vi "PH_DIM.get String.vi"(1 "no link":bool, 2 "typeDescriptor":string, 3 "data":i8[](array[numeric]), 4 "quality":i32) -> (0 "Output String":string)   [LabVIEW 2014, in "PH_Common.lvlib"]
doc: "This VI calculates the status of a string tag. It gives out:\n\nno info available: no link or wrong data type or tag status bad\nelse: link and data type and tag status ok, value = incoming text"
uses:
  PH_Common.lvlib
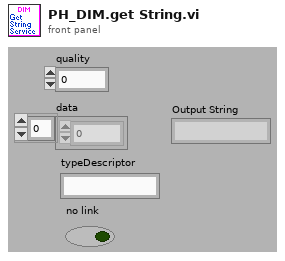
[diagram p1: front panel]
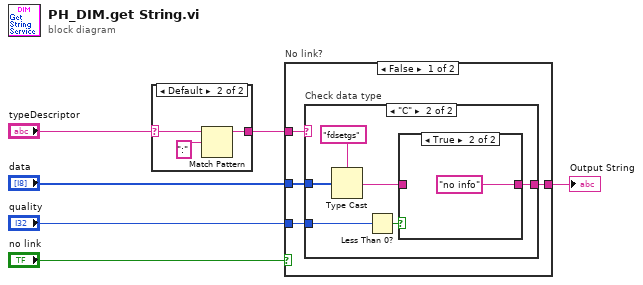
[diagram p0: block diagram]
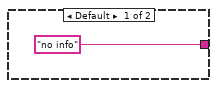
[diagram p3: hidden frame]
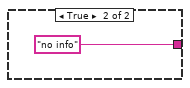
[diagram p5: hidden frame]
diagram:
  n1 = case shown="Default" "typeDescriptor" {
    selector: "typeDescriptor" -> [w7 w8]
    tunnel: [w7 w10] -> w2
    frame "C" {
    }
    frame Default {
      n2 = Match Pattern(string=w8, regular expression=":") -> (before substring=w10:string)  [unwired: 1 in, 3 out]
    }
  }
  n3 = case "No link?" shown="False" "no link" {
    tunnel: [w14 "no info"] -> w6
    tunnel: "quality" -> [w13 _]
    tunnel: "data" -> [w12 _]
    tunnel: w2 -> [w11 _]
    frame False {
      n4 = case "Check data type" shown="\"C\"" w11 {
        tunnel: ["no info" w21] -> w14
        tunnel: w13 -> [_ w19]
        tunnel: w12 -> [_ w18]
        frame Default {
        }
        frame "C" {
          n5 = Type Cast(type="fdsetgs", x=w18) -> (*(type *) &x=w17:string)
          n6 = Less Than 0?(x=w19) -> (x < 0?=w20:bool)
          n7 = case shown="True" w20 {
            tunnel: [w22 "no info"] -> w21
            tunnel: w17 -> [w22 _]
            frame False {
            }
            frame True {
            }
          }
        }
      }
    }
    frame True {
    }
  }
  "Output String" <- w6
